vi "LogCfg.vi"(0 "SamplesIn":i32=1000 caption="No of Samples" min=2, 1 "FastIn":bool caption="Fast Logging to File\n(w/o display update)", 2 "PM16":bool, 5 "IntervalIn":dbl=1.0 caption="Interval Time [s]" min=0.1 max=9999.9 step=0.1 format="%.1f", 7 "ACCON":bool, 9 "AveragingIn":i32=100 caption="Averaging" min=1 max=100 step=1, 11 "FileIn":bool caption="Select Log File", 12 "SensType":i32(ring) items=["No Sensor", "Photo", "Thermo", "Pyro"], 14 "LogPath":path) -> (3 "FileRefnum":refnum<file>, 4 "SamplesOut":i32, 6 "IntervalOut":dbl, 10 "AveragingOut":i32, 13 "FastOut":bool, 15 "FileOut":bool)   [LabVIEW 2011]
panel:
  out "days":i16
  out "hh":i16
  out "mm":i16
  out "ss":i16
  out "Est Tm":dbl
  out "error out":errorcluster
  in  "stop":bool
  # "Configure Data Logging"
  # "- No of Samples\n- Averaging Rate\n- Interval\n- File"
  # "Duration"
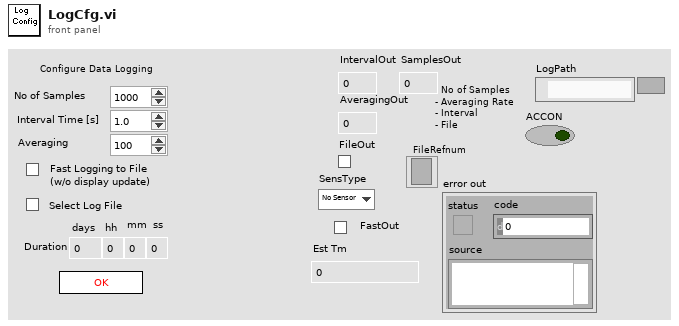
[diagram p1: front panel]
types:
  T1 = enum16{"open", "replace", "create", "open or create", "replace or create", "replace or create with confirmation"}
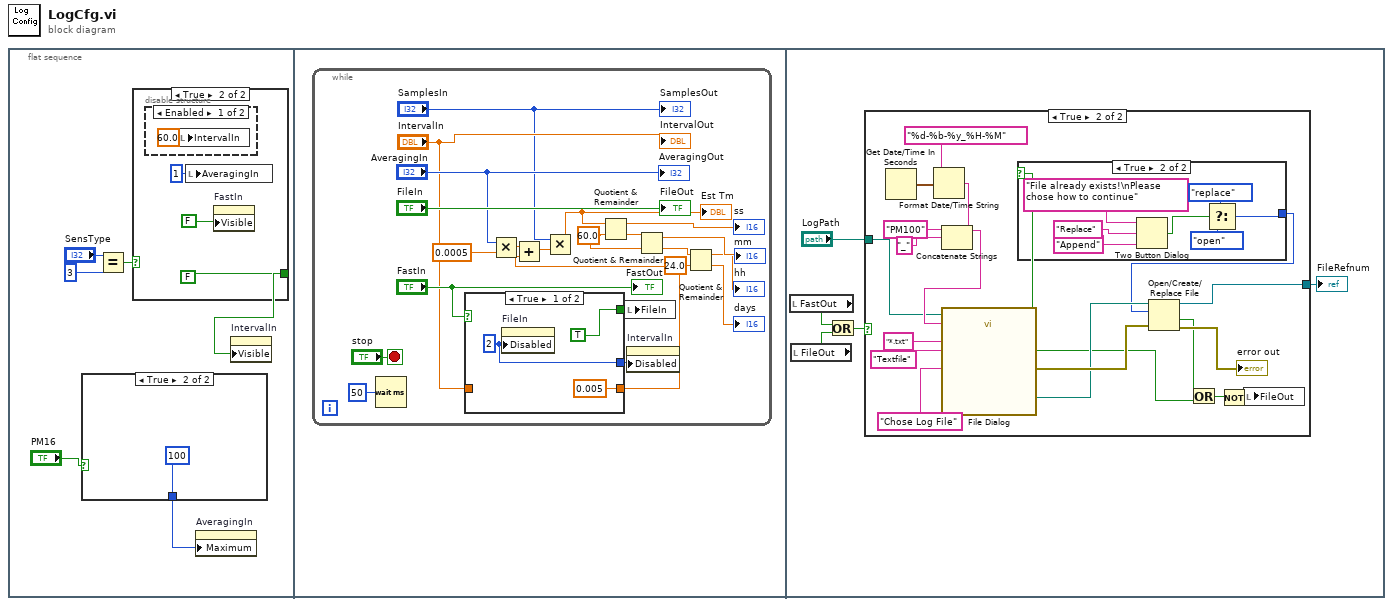
[diagram p0: block diagram]
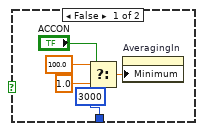
[diagram p2: hidden frame]
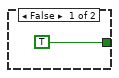
[diagram p3: hidden frame]
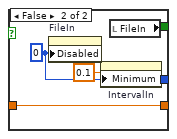
[diagram p5: hidden frame]
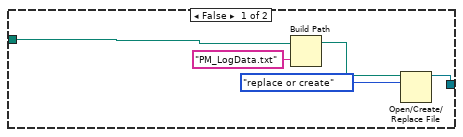
[diagram p6: hidden frame]
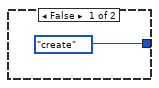
[diagram p7: hidden frame]
diagram:
  n1 = flat-sequence {
    frame #0 {
      n2 = case shown="True" "PM16" {
        tunnel: [3000 100] -> w1
        frame False {
          n3 = Select(t=100.0, s="ACCON", f=1.0) -> (s? t:f=w11:dbl)
          n4 = property on="AveragingIn" class="DigNum (strict)"("Minimum"=w11) -> ()  [unwired: 2 in, 2 out]
        }
        frame True {
        }
      }
      n5 = Equal?(x="SensType", y=3) -> (x = y?=w4:bool)
      n6 = case shown="True" w4 {
        tunnel: [TRUE ("Visible") FALSE ("Visible")] -> w3
        frame False {
        }
        frame True {
          n7 = disable-structure shown="Enabled" {
            frame Enabled {
              n8 = local write "IntervalIn"(60.0 ("IntervalIn")) -> ()
            }
            frame Disabled {
            }
          }
          n9 = local write "AveragingIn"(1 ("AveragingIn")) -> ()
          n10 = property on="FastIn" class="Bool (strict)"("Visible"=FALSE) -> ()  [unwired: 2 in, 2 out]
        }
      }
      n11 = property on="AveragingIn" class="DigNum (strict)"("Maximum"=w1) -> ()  [unwired: 2 in, 2 out]
      n12 = property on="IntervalIn" class="DigNum (strict)"("Visible"=w3) -> ()  [unwired: 2 in, 2 out]
    }
    frame #1 {
      n13 = while {
        stop <- "stop" stop-if-true
        w23 = 60.0 ("y")
        n14 = Wait (ms)(milliseconds to wait=u32 50) -> ()  [unwired: 1 out]
        n15 = case shown="True" "FastIn" {
          tunnel: [TRUE w46] -> w35
          tunnel: [w41 w45] -> w34
          tunnel: [0.005 ("IntervalIn") w43] -> w29
          tunnel: "IntervalIn" -> [_ w43]
          frame True {
            w41 = u8 2 ("Disabled")
            n16 = property on="FileIn" class="Bool (strict)"("Disabled"=w41) -> ()  [unwired: 2 in, 2 out]
          }
          frame False {
            w45 = u8 0 ("Disabled")
            n17 = property on="FileIn" class="Bool (strict)"("Disabled"=w45) -> ()  [unwired: 2 in, 2 out]
            n18 = property on="IntervalIn" class="DigNum (strict)"("Minimum"=0.1 ("Data Entry Limits:Minimum")) -> ()  [unwired: 2 in, 2 out]
            n19 = local read "FileIn"() -> (w46:bool)
          }
        }
        n20 = Multiply(x="AveragingIn", y=0.0005 ("Data Entry Limits:Minimum")) -> (x*y=w30:dbl)
        n21 = Add(x=w30, y=w29) -> (x+y=w28:dbl)
        n22 = Multiply(x="SamplesIn", y=w28) -> (x*y=w26:dbl)
        "Est Tm" <- w26
        n23 = Quotient & Remainder(x=w26, y=w23) -> (x-y*floor(x/y)=→"ss":dbl, floor(x/y)=w24:dbl)
        n24 = local write "FileIn"(w35) -> ()
        n25 = property on="IntervalIn" class="DigNum (strict)"("Disabled"=w34) -> ()  [unwired: 2 in, 2 out]
        n26 = Quotient & Remainder(x=w24, y=w23) -> (x-y*floor(x/y)=→"mm":dbl, floor(x/y)=w21:dbl)
        n27 = Quotient & Remainder(x=w21, y=24.0) -> (x-y*floor(x/y)=→"hh":dbl, floor(x/y)=→"days":dbl)
        "IntervalOut" <- "IntervalIn"
        "SamplesOut" <- "SamplesIn"
        "AveragingOut" <- "AveragingIn"
        "FileOut" <- "FileIn"
        "FastOut" <- "FastIn"
      }
    }
    frame #2 {
      n28 = local read "FastOut"() -> (w50:bool)
      n29 = local read "FileOut"() -> (w49:bool)
      n30 = Or(x=w50, y=w49) -> (x .or. y?=w51:bool)
      n31 = case shown="True" w51 {
        tunnel: [w56 w58] -> w48
        tunnel: "LogPath" -> [w52 w57]
        frame False {
          n32 = Build Path(base path=w52, name or relative path="PM_LogData.txt") -> (appended path=w53:path)
          n33 = Open/Create/Replace File(file path (use dialog)=w53, operation (0:open)=T1."replace or create") -> (refnum out=w56:refnum<file>)  [unwired: 4 in, 2 out]
        }
        frame True {
          n34 = Get Date/Time In Seconds() -> (seconds since 1Jan1904=w64:timestamp)
          n35 = Format Date/Time String(time format string (%c)="%d-%b-%y_%H-%M", seconds (now)=w64) -> (date/time string=w61:string)  [unwired: 1 in]
          n36 = Concatenate Strings("PM100" ("default name"), "_" ("string"), w61) -> (w65:string)
          n37 = call "File Dialog"("start path"=w57, "prompt"="Chose Log File", "default name"=w65, "pattern (all files)"="*.txt", "pattern label"="Textfile" ("button label")) -> ("selected path"=w73:path, "exists"=w60:bool, "cancelled"=w69:bool, "error out"=w74:errorcluster)  [unwired: 7 in]
          n38 = case shown="True" w60 {
            tunnel: [T1."create" ("operation (0:open)") w78] -> w59
            frame False {
            }
            frame True {
              n39 = Two Button Dialog(message="File already exists!\nPlease chose how to continue", 1:"Append" ("F button name (\"Cancel\")"), 2:"Replace" ("T button name (\"OK\")")) -> (T button?=w80:bool)
              n40 = Select(t=T1."replace" ("operation (0:open)"), s=w80, f=T1."open" ("operation (0:open)")) -> (s? t:f=w78:T1)
            }
          }
          n41 = Open/Create/Replace File(file path (use dialog)=w73, error in=w74, operation (0:open)=w59) -> (refnum out=w58:refnum<file>, cancelled=w67:bool, error out=→"error out":errorcluster)  [unwired: 3 in]
          n42 = Or(x=w67, y=w69) -> (x .or. y?=w68:bool)
          n43 = Not(x=w68) -> (.not. x?=w76:bool)
          n44 = local write "FileOut"(w76) -> ()
        }
      }
      "FileRefnum" <- w48
    }
  }
